vi "Gait to Desired Theta.vi"(11 "Current Gait %":dbl) -> (2 "Current Desired Theta":dbl)   [LabVIEW 2018]
uses:
  <vilib>/Simulation/Scripting/Companion Diagram/SimConfigNode/SimParams.ctl
  <vilib>/Simulation/Scripting/Companion Diagram/SimConfigNode/_simSolvers.ctl
  <vilib>/Simulation/Implementation/Shared/SIMSCR Execution Mode.ctl
  <vilib>/Simulation/Param Hierarchy/Typedefs/SIMPH Param Control Actions.ctl
  <vilib>/Simulation/Implementation/Shared/NILVSim_ParamChanged.vi
  <vilib>/Simulation/Implementation/Shared/NILVSIM_BeginStep.vi
  <vilib>/Simulation/LookUpTables/Implementation/NILVSim LUT 1D.llb/SIM LUT 1D (scalar).vi
  <vilib>/Simulation/Implementation/Shared/NILVSim_Manager.vi
  <vilib>/Utility/error.llb/Clear Errors.vi
  <vilib>/Simulation/Implementation/Shared/NILVSim_FinalizeModel.vi
  <vilib>/Simulation/Implementation/Shared/SIM Unbundle Sim Info.vi
  <vilib>/Simulation/Implementation/Shared/NILVSim_Initialize.vi
  <vilib>/Simulation/Utility/Implementation/NILVSim Get Time and IsAcceptedStep.vi
  <vilib>/Simulation/Implementation/Shared/SIMSH Read Queue.vi
  <vilib>/Simulation/Implementation/Shared/NILVSim_GetModelError.vi
  <vilib>/Simulation/Implementation/Shared/SIM Bundle Sim Info.vi
  <vilib>/Simulation/Scripting/Companion Diagram/SimConfigNode/SimDog.xnode
  <vilib>/Simulation/Implementation/XNodeFramework/SimXNode/SimX.xnode
  <vilib>/gmath/NI_Gmath.lvlib
  <vilib>/Simulation/Implementation/Shared/NI_SIM_Implementation.lvlib
panel:
  out "LUT Results 2":dbl(graph)
  out "Desired Kinematic Trajectory":cluster{"Ramp Pattern":dbl[], "first row":dbl[]}(graph)
  out "ILC theta_d":dbl[](array[numeric])
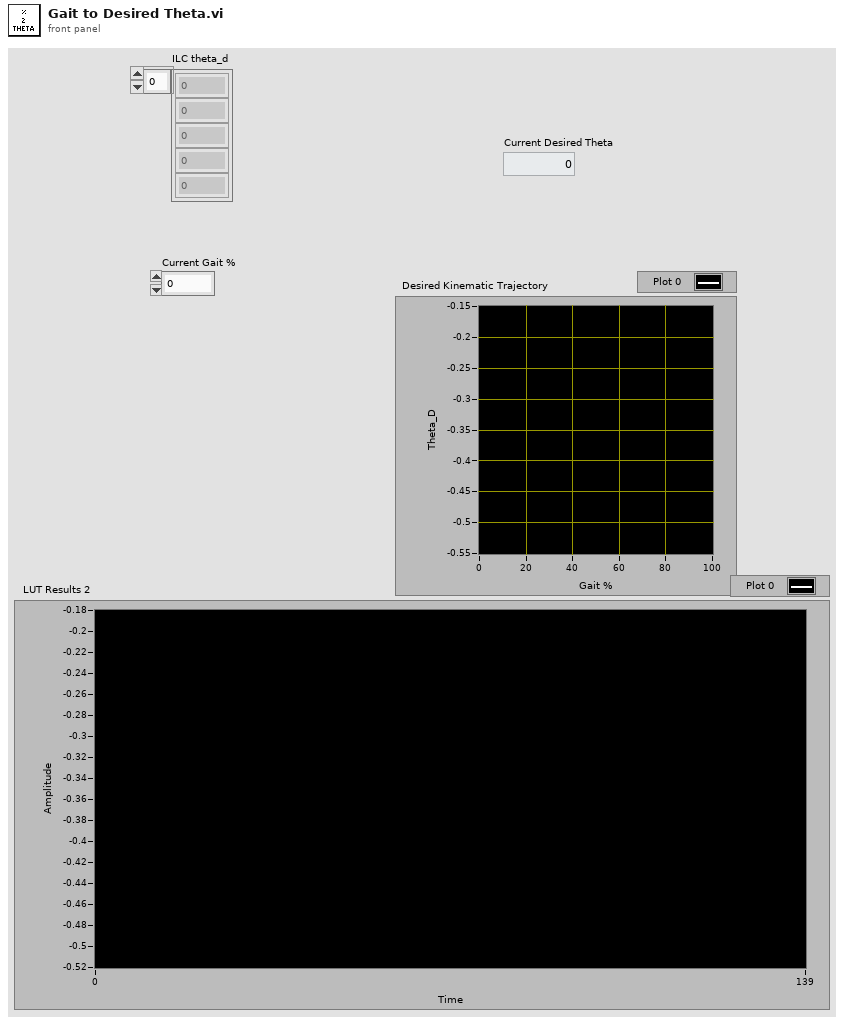
[diagram p1: front panel]
types:
  T1 = cluster{"Array of Double":dbl[], "Array of Double":dbl[]}
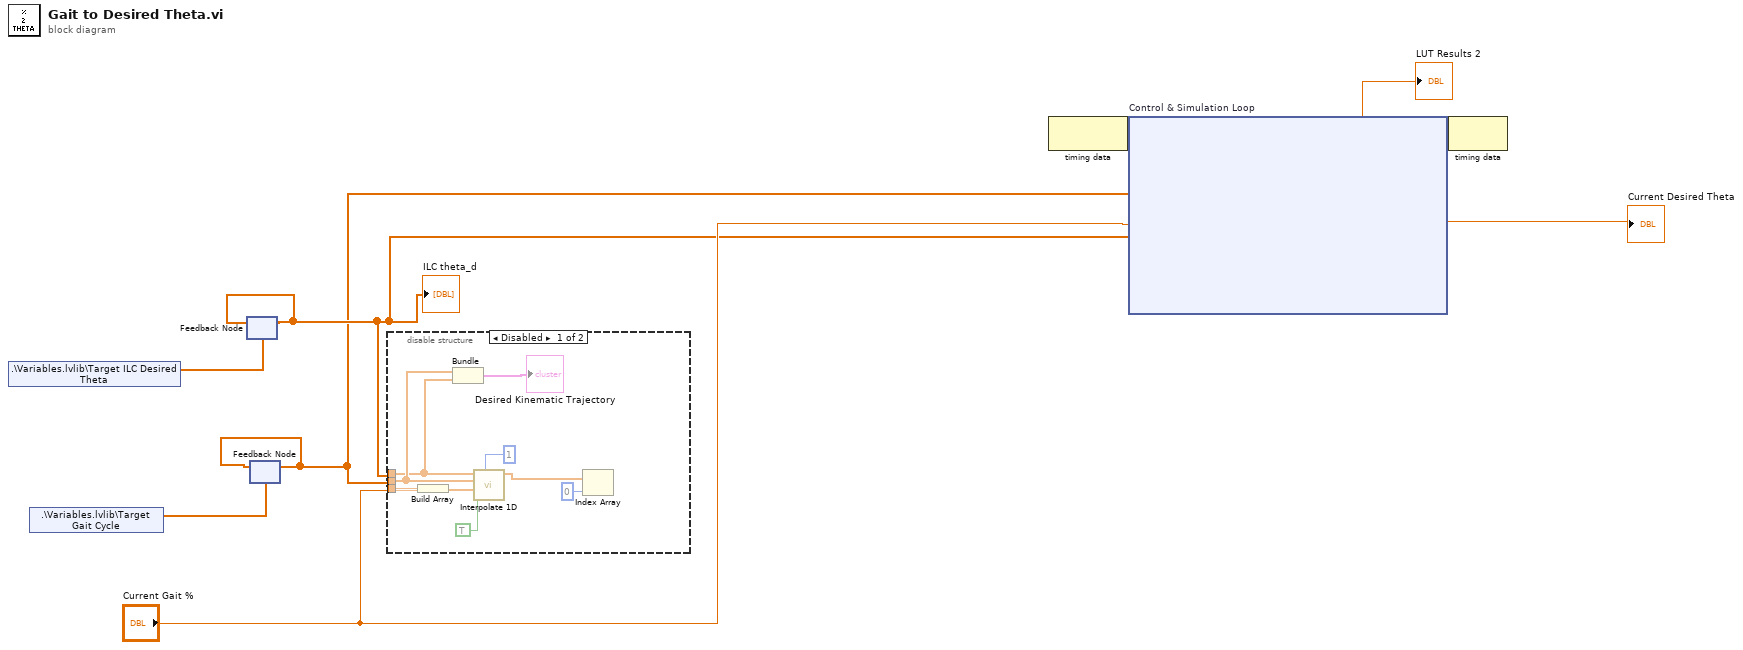
[diagram p0: block diagram]
diagram:
  n1 = shared-variable ".\\Variables.lvlib\\Target ILC Desired Theta"() -> (w4:dbl[])  [unwired: 1 in, 1 out]
  n2 = shared-variable ".\\Variables.lvlib\\Target Gait Cycle"() -> (w2:dbl[])  [unwired: 1 in, 1 out]
  n3 = feedback #1(w4) -> (w3:dbl[])
  "ILC theta_d" <- w3
  n4 = feedback-in #1(w3) -> ()
  n5 = feedback #2(w2) -> (w1:dbl[])
  n6 = feedback-in #2(w1) -> ()
  n7 = disable-structure shown="Disabled" {
    disable-tunnel: "Current Gait %" -> [w14 _]
    disable-tunnel: w1 -> [w11 _]
    disable-tunnel: w3 -> [w10 _]
    frame Disabled {
      n8 = Build Array(w14) -> (w13:dbl[])
      n9 = Bundle("Array of Double"=w11, "Array of Double"=w10) -> (→"Desired Kinematic Trajectory":T1)  [unwired: 1 in]
      n10 = call <vilib>:"Interpolate 1D.vi"("method"=1, "X is monotonic"=TRUE, "xi"=w13, "X"=w11, "Y"=w10) -> ("yi"=w16:dbl[])  [unwired: 4 in, 2 out]
      n11 = Index Array(array=w16, index=0) -> ()  [unwired: 1 out]
    }
    frame Enabled {
    }
  }
  n12 = node-c288() -> (w9:variant)  [unwired: 1 in]
  n13 = node-c254 "Control & Simulation Loop"(w9, w3, w1, "Current Gait %") -> (w8:variant, →"LUT Results 2":dbl, →"Current Desired Theta":dbl)
  n14 = node-c288(w8) -> ()  [unwired: 1 out]
